vi "Teleop.vi"(10 "Match Info":T1={"Autonomous Elapsed Seconds"=0.0, "TeleOp Elapsed Seconds"=0.0, "Disabled Elapsed Seconds"=0.0, "Visited Autonomous"=FALSE, "Visited TeleOp"=FALSE, "Visited Disabled"=FALSE, "Autonomous Settings"={"Autonomous Style"=enum."Independent", "VI Refnum"=refnum}}, 11 "Call Context":T2) -> ()   [LabVIEW 2020]
doc: "This VI is called for each TeleOp packet received from the DS where the robot is not disabled. It is often used to read from the joysticks and update I/O or to update setpoints for timed control loops. It should complete and return within 20 milliseconds or it may miss DS packets."
uses:
  <vilib>/Rock Robotics/WPI/DriverStation/WPI_DriverStationDerivedRobotMode.ctl
  <vilib>/Rock Robotics/WPI/DriverStation/WPI_DriverStationMatch Info.ctl
  <vilib>/Rock Robotics/WPI/ThirdParty/Phoenix-LabVIEW/Motor Controller/Controls/CTRE_Phoenix_MotorControl_ControlMode.ctl
  <vilib>/Rock Robotics/WPI/ThirdParty/Phoenix-LabVIEW/Controls/CTRE_Phoenix_Params.ctl
  <vilib>/Rock Robotics/WPI/Utilities/WPI_GetSetVariantRefNum.vi
  <vilib>/Rock Robotics/Network Tables/NT Write Boolean Array.vi
  <vilib>/Rock Robotics/Network Tables/NT Write Numeric Array.vi
  <vilib>/Rock Robotics/Network Tables/NT Read Boolean.vi
  <vilib>/Rock Robotics/Network Tables/NT Read Number.vi
  <vilib>/Rock Robotics/WPI/Solenoid/Deprecated/WPI_SolenoidSetBool.vi
panel:
  out "encoder value":dbl
  out "Sample Slider 0":dbl(slide) scale=0.0..5.0
  out "Sample Boolean 1":bool
  out "Sample Boolean 0":bool
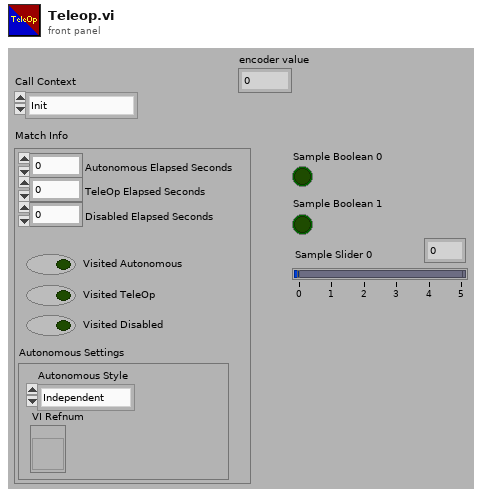
[diagram p1: front panel]
types:
  T1 = typedef "WPI_DriverStationMatch Info.ctl" = cluster{"Autonomous Elapsed Seconds":dbl, "TeleOp Elapsed Seconds":dbl, "Disabled Elapsed Seconds":dbl, "Visited Autonomous":bool, "Visited TeleOp":bool, "Visited Disabled":bool, "Autonomous Settings":cluster{"Autonomous Style":enum16{"Iterative", "Independent"}, "VI Refnum":refnum<vi>}}
  T2 = typedef "WPI_DriverStationDerivedRobotMode.ctl" = enum16{"Init", "Execute", "Stop"}
  T3 = typedef "CTRE_Phoenix_Params.ctl" = u16
  T4 = typedef "CTRE_Phoenix_MotorControl_ControlMode.ctl" = u16
  T5 = typedef "WPI_MotorControlDeviceRef.ctl" = cluster{"DeviceStatus":errorcluster, "Type":T6, "PWM":cluster{"PWM Channel":T7, "DeadBand":T8}, "CAN":cluster{"Device Number":u8, "SetOutput VI Ref":variant, "GetOutput VI Ref":variant, "Enable VI Ref":variant, "Disable VI Ref":variant, "Data":variant}, "Invert":bool, "DIO PWM":cluster{"PWM \"Enable\" Channel":T7, "DIOChannel":T9, "PWM Rate":dbl}}
  T6 = typedef "WPI_MotorControlType.ctl" = enum16{"PWM", "CAN", "DIO PWM"}
  T7 = typedef "FPGA_DIOPWMChannel.ctl" = enum8{"PWM 0", "PWM 1", "PWM 2", "PWM 3", "PWM 4", "PWM 5", "PWM 6", "PWM 7", "PWM 8", "PWM 9", "PWM MXP 0", "PWM MXP 1", "PWM MXP 2", "PWM MXP 3", "PWM MXP 4", "PWM MXP 5", "PWM MXP 6", "PWM MXP 7", "PWM MXP 8", "PWM MXP 9", "Invalid"}
  T8 = typedef "WPI_PWMDeadband.ctl" = cluster{"Name":string, "maxPositivePwm":i32, "minPositivePwm":i32, "centerPwm":i32, "maxNegativePwm":i32, "minNegativePwm":i32, "angularRange":u16}
  T9 = typedef "FPGA_DIOChannel.ctl" = enum8{"DIO 0", "DIO 1", "DIO 2", "DIO 3", "DIO 4", "DIO 5", "DIO 6", "DIO 7", "DIO 8", "DIO 9", "DIO MXP 0", "DIO MXP 1", "DIO MXP 2", "DIO MXP 3", "DIO MXP 4", "DIO MXP 5", "DIO MXP 6", "DIO MXP 7", "DIO MXP 8", "DIO MXP 9", "DIO MXP 10", "DIO MXP 11", "DIO MXP 12", "DIO MXP 13", "DIO MXP 14", "DIO MXP 15", "SPI Port CS1", "SPI Port CS2", "SPI Port CS3", "SPI Port MISO", "SPI Port MOSI", "Invalid"}
  T10 = typedef "WPI_JoystickDevRef.ctl" = cluster{"Device":T11}
  T11 = typedef "WPI_JoystickDeviceEnum.ctl" = enum16{"USB 0", "USB 1", "USB 2", "USB 3", "USB 4", "USB 5"}
  T12 = cluster{"Buttons[0]":bool, "Buttons[1]":bool, "Buttons[2]":bool, "Buttons[3]":bool, "Buttons[4]":bool, "Buttons[5]":bool, "Buttons[6]":bool, "Buttons[7]":bool, "Buttons[8]":bool}
  T13 = cluster{"Axes[0]":dbl, "Axes[1]":dbl, "Axes[2]":dbl, "Axes[3]":dbl, "Axes[4]":dbl, "Axes[5]":dbl, "Axes[6]":dbl, "Axes[7]":dbl, "Axes[8]":dbl}
  T14 = typedef "WPI_RobotDriveDevRef.ctl" = cluster{"DevStatus":errorcluster, "Motors[]":T5[], "Square Inputs":bool, "Max Output":dbl}
  T15 = typedef "WPI_SolenoidDevRef.ctl" = cluster{"DevStatus":errorcluster, "Pneumatics Control Module":u8, "Forward Solenoid Channel":T16, "Reverse Solenoid Channel":T16}
  T16 = typedef "WPI_SolenoidChannel.ctl" = enum8{"Solenoid 0", "Solenoid 1", "Solenoid 2", "Solenoid 3", "Solenoid 4", "Solenoid 5", "Solenoid 6", "Solenoid 7", "Solenoid 8", "Solenoid 9", "Solenoid 10", "Solenoid 11", "Solenoid 12", "Solenoid 13", "Solenoid 14", "Solenoid 15", "Invalid"}
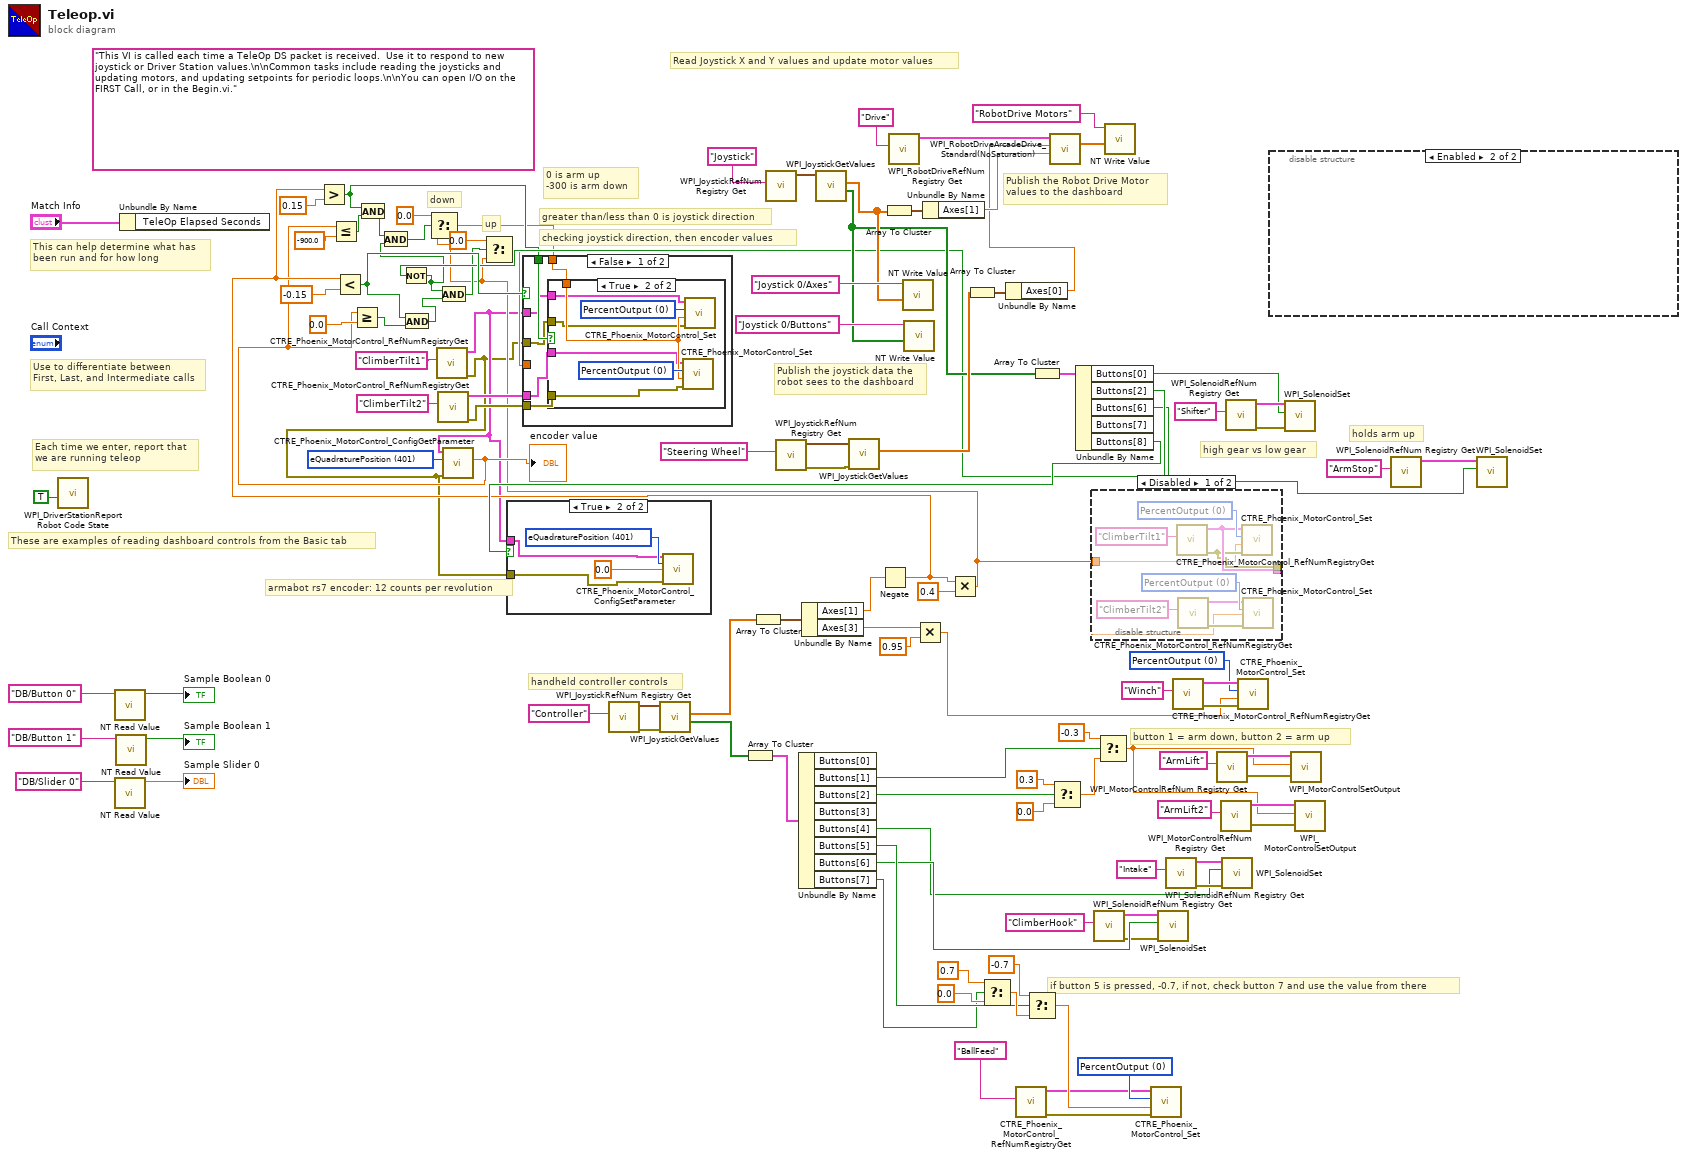
[diagram p0: block diagram]
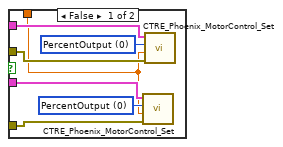
[diagram p3: hidden frame]
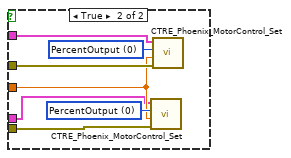
[diagram p4: hidden frame]
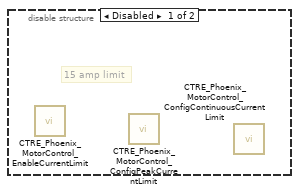
[diagram p6: hidden frame]
diagram:
  w22 = T3 401 items=["eOnBoot_BrakeMode"=31, "eQuadFilterEn"=91, "eClearPositionOnIdx"=100, "eQuadIdxPolarity"=108, "eMotionProfileHasUnderrunErr"=119, "eMotionProfileTrajectoryPointDurationMs"=120, "eMotionProfileTrajectoryInterpolDis"=121, "eClearPosOnLimitF"=144, "eClearPosOnLimitR"=145, "eYawOffset"=160, "eCompassOffset"=161, "eBetaGain"=162, "eEnableCompassFustion"=163, "eGyroNoMotionCal"=164, "eEnterCalibration"=165, "eFusedHeadingOffset"=166, "eStatusFrameRate"=169, "eAccumZ"=170, "eTempCompDisable"=171, "eMotionMeas_tap_threshX"=172, "eMotionMeas_tap_threshY"=173, "eMotionMeas_tap_threshZ"=174, "eMotionMeas_tap_count"=175, "eMotionMeas_tap_time"=176, "eMotionMeas_tap_time_multi"=177, "eMotionMeas_shake_reject_thresh"=178, "eMotionMeas_shake_reject_time"=179, "eMotionMeas_shake_reject_timeout"=180, "eStatusFramePeriod"=300, "eOpenLoopRamp"=301, "eClosedLoopRamp"=302, "eNeutralDeadband"=303, "ePeakPosOutput"=305, "eNominalPosOutput"=306, "ePeakNegOutput"=307, "eNominalNegOutput"=308, "eProfileParamSlot_P"=310, "eProfileParamSlot_I"=311, "eProfileParamSlot_D"=312, "eProfileParamSlot_F"=313, "eProfileParamSlot_IZone"=314, "eProfileParamSlot_AllowableErr"=315, "eProfileParamSlot_MaxIAccum"=316, "eProfileParamSlot_PeakOutput"=317, "eClearPositionOnLimitF"=320, "eClearPositionOnLimitR"=321, "eClearPositionOnQuadIdx"=322, "eSampleVelocityPeriod"=325, "eSampleVelocityWindow"=326, "eFeedbackSensorType"=330, "eSelectedSensorPosition"=331, "eFeedbackNotContinuous"=332, "eRemoteSensorSource"=333, "eRemoteSensorDeviceID"=334, "eSensorTerm"=335, "eRemoteSensorClosedLoopDisableNeutralOnLOS"=336, "ePIDLoopPolarity"=337, "ePIDLoopPeriod"=338, "eSelectedSensorCoefficient"=339, "eForwardSoftLimitThreshold"=340, "eReverseSoftLimitThreshold"=341, "eForwardSoftLimitEnable"=342, "eReverseSoftLimitEnable"=343, "eNominalBatteryVoltage"=350, "eBatterVoltageFilterSize"=351, "eContinuousCurrentLimitAmps"=360, "eContinuousCurrentLimitMs"=361, "ePeakCurrentLimitAmps"=362, "eCurrEnable"=363, "eCurrThres_Ms"=364, "eClosedLoopIAccum"=370, "eCustomParam"=380, "eStickyFaults"=390, "eAnalogPosition"=400, "eQuadraturePosition"=401, "ePulseWidthPosition"=402, "eIntegratedSensor"=403, "eMotMag_Accel"=410, "eMotMag_VelCruise"=411, "eMotMag_SCurveLevel"=412, "eLimitSwitchSource"=421, "eLimitSwitchNormClosedAndDis"=422, "eLimitSwitchDisabledNeutralOnLOS"=423, "eLimitSwitchRemoteDevID"=424, "eSoftLimitDisabledNeutralOnLOS"=425, "ePulseWidthPeriod_EdgesPerRot"=430, "ePulseWidthPeriod_FilterWindowSz"=431, "eUnitString"=442, "eFeedbackTimeBase"=443, "eDefaultConfig"=500, "eFastWriteCount"=501, "eWriteCount"=502, "eReserved1"=555, "eMotorCommutation"=650, "eSensorInitStrategy"=700, "eSensorDirection"=701, "eMagnetOffset"=702, "eSensorSync"=703, "eAbsSensorRange"=704, "eChangeCompassUse"=800, "eRestartKalman"=801, "eAccNoiseAmplificationGain"=802, "eMagNoiseAmplificationGain"=803, "eGyrNoiseAmplificationGain"=804, "eMaxAccKg"=805, "eMaxMagKg"=806, "eGyroBias"=807, "eAccelOffsets"=808, "eMagCal"=809, "eMagCalSlot"=810, "eMagCalRunning"=811, "eGyrResolution"=812, "eAccelKalmanBiasGain"=813, "eMagKalmanBiasGain"=814, "eTempCalRunning"=815, "eApplyTempCal"=816, "eClearTempCal"=817, "eDontRunThermComp"=818, "eChangeHeatOutput"=819, "eSetNoMotionCalDisable"=820, "eClearMagCal"=821, "eSetGyrSensitivity"=822, "eSetVsenseScalar"=823, "eConfigMountPoseYaw"=824, "eConfigMountPosePitch"=825, "eConfigMountPoseRoll"=826, "eConfigAccelScalar"=827, "eLEDStripType"=900, "eLossOfSignalBehavior"=901, "eBrightnessCoefficient"=902, "eStatusLedState"=903, "eVBatOutput"=904] ("Parameter")
  w48 = T4 0 items=["PercentOutput"=0, "Position"=1, "Velocity"=2, "Current"=3, "Follower"=5, "MotionProfile"=6, "MotionMagic"=7, "MotionProfileArc"=10, "Disabled"=15] ("Control Mode")
  w79 = T4 0 items=["PercentOutput"=0, "Position"=1, "Velocity"=2, "Current"=3, "Follower"=5, "MotionProfile"=6, "MotionMagic"=7, "MotionProfileArc"=10, "Disabled"=15] ("Control Mode")
  (unwired) "This VI is called each time a TeleOp DS packet is received.  Use it to respond to new joystick or Driver Station values.\n\nCommon tasks include reading the joysticks and updating motors, and updating setpoints for periodic loops.\n\nYou can open I/O on the FIRST Call, or in the Begin.vi."
  # "down"
  # "up"
  # "checking joystick direction, then encoder values"
  # "greater than/less than 0 is joystick direction"
  # "0 is arm up\n-300 is arm down"
  # "armabot rs7 encoder: 12 counts per revolution"
  # "holds arm up"
  # "button 1 = arm down, button 2 = arm up"
  # "if button 5 is pressed, -0.7, if not, check button 7 and use the value from there"
  # "high gear vs low gear"
  # "handheld controller controls"
  # "These are examples of reading dashboard controls from the Basic tab"
  # "Publish the Robot Drive Motor\nvalues to the dashboard"
  # "Publish the joystick data the\nrobot sees to the dashboard"
  # "Each time we enter, report that\nwe are running teleop"
  # "Use to differentiate between\nFirst, Last, and Intermediate calls"
  # "This can help determine what has\nbeen run and for how long"
  # "Read Joystick X and Y values and update motor values"
  n1 = call <vilib>:"WPI_DriverStationReport Robot Code State.vi"("TeleOp"=TRUE ("Autonomous")) -> ()  [unwired: 10 in, 1 out]
  n2 = call-poly <vilib>:"NT Read Value.vi"("Name"="DB/Button 0" ("refnum name")) -> ("Boolean"=→"Sample Boolean 0":bool)  [unwired: 9 in, 1 out]
  n3 = call-poly <vilib>:"NT Read Value.vi"("Name"="DB/Slider 0" ("refnum name")) -> ("Numeric"=→"Sample Slider 0":dbl)  [unwired: 9 in, 1 out]
  n4 = call-poly <vilib>:"NT Read Value.vi"("Name"="DB/Button 1" ("refnum name")) -> ("Boolean"=→"Sample Boolean 1":bool)  [unwired: 9 in, 1 out]
  n5 = Unbundle By Name("Match Info") -> ()  [unwired: 1 out]
  n6 = call <vilib>:"CTRE_Phoenix_MotorControl_RefNumRegistryGet.vi"("refnum name"="ClimberTilt1") -> ("error out"=w1:errorcluster, "PhoenixMotorControlDevRef"=w2:T5)  [unwired: 9 in]
  n7 = call <vilib>:"CTRE_Phoenix_MotorControl_RefNumRegistryGet.vi"("refnum name"="ClimberTilt2") -> ("error out"=w20:errorcluster, "PhoenixMotorControlDevRef"=w21:T5)  [unwired: 9 in]
  n8 = call <vilib>:"CTRE_Phoenix_MotorControl_ConfigGetParameter.vi"("error in (no error)"=w1, "Parameter"=w22, "PhoenixMotorControlDevRef"=w2) -> ("value"=w15:dbl)  [unwired: 6 in, 2 out]
  "encoder value" <- w15
  n9 = Less Or Equal?(x=w15, y=-900.0) -> (x <= y?=w12:bool)
  n10 = Greater Or Equal?(x=w15, y=0.0) -> (x >= y?=w26:bool)
  n11 = call <vilib>:"WPI_JoystickRefNum Registry Get.vi"("refnum name"="Controller") -> ("error out"=w86:errorcluster, "JoystickDevRef"=w85:T10)  [unwired: 9 in]
  n12 = call <vilib>:"WPI_JoystickGetValues.vi"("error in (no error)"=w86, "JoystickDevRef"=w85) -> ("Buttons"=w83:bool[], "Axes"=w70:dbl[])  [unwired: 5 in, 3 out]
  n13 = Array To Cluster(array=w83) -> (cluster=w82:T12)
  n14 = Array To Cluster(array=w70) -> (cluster=w69:T13)
  n15 = call <vilib>:"WPI_JoystickRefNum Registry Get.vi"("refnum name"="Joystick") -> ("JoystickDevRef"=w107:T10)  [unwired: 1 in, 9 out]
  n16 = call <vilib>:"WPI_JoystickRefNum Registry Get.vi"("refnum name"="Steering Wheel") -> ("error out"=w94:errorcluster, "JoystickDevRef"=w95:T10)  [unwired: 9 in]
  n17 = Unbundle By Name(w82) -> ("Buttons[1]"=w68:bool, "Buttons[2]"=w66:bool, "Buttons[4]"=w39:bool, "Buttons[5]"=w59:bool, "Buttons[6]"=w43:bool, "Buttons[7]"=w58:bool)  [unwired: 2 out]
  n18 = Unbundle By Name(w69) -> ("Axes[1]"=w33:dbl, "Axes[3]"=w46:dbl)
  n19 = call <vilib>:"WPI_JoystickGetValues.vi"("JoystickDevRef"=w107) -> ("Buttons"=w57:bool[], "Axes"=w92:dbl[])  [unwired: 6 in, 3 out]
  n20 = call <vilib>:"WPI_JoystickGetValues.vi"("error in (no error)"=w94, "JoystickDevRef"=w95) -> ("Axes"=w90:dbl[])  [unwired: 5 in, 4 out]
  n21 = Negate(x=w33) -> (-x=w17:dbl)
  n22 = Greater?(x=w17, y=0.15) -> (0:w13:bool)
  n23 = Less?(x=w17, y=-0.15) -> (x < y?=w19:bool)
  n24 = And(x=w13, y=w12) -> (x .and. y?=w11:bool)
  n25 = And(x=w19, y=w26) -> (x .and. y?=w25:bool)
  n26 = Array To Cluster(array=w92) -> (cluster=w91:T13)
  n27 = call <vilib>:"WPI_RobotDriveRefNum Registry Get.vi"("refnum name"="Drive") -> ("RobotDriveDevRef"=w109:T14)  [unwired: 1 in, 9 out]
  n28 = call-poly <vilib>:"NT Write Value.vi"("Numeric Array"=w92, "Name"="Joystick 0/Axes") -> ()  [unwired: 9 in, 1 out]
  n29 = call-poly <vilib>:"NT Write Value.vi"("Boolean Array"=w57, "Name"="Joystick 0/Buttons") -> ()  [unwired: 9 in, 1 out]
  n30 = Multiply(x=w46, y=0.95) -> (x*y=w44:dbl)
  n31 = Unbundle By Name(w91) -> ("Axes[1]"=w88:dbl)
  n32 = Multiply(x=w17, y=0.4) -> (x*y=w4:dbl)
  n33 = Array To Cluster(array=w90) -> (cluster=w89:T13)
  n34 = Select(t=0.7, s=w58, f=0.0) -> (s? t:f=w77:dbl)
  n35 = Unbundle By Name(w89) -> ("Axes[0]"=w87:dbl)
  n36 = call <vilib>:"CTRE_Phoenix_MotorControl_RefNumRegistryGet.vi"("refnum name"="BallFeed") -> ("error out"=w74:errorcluster, "PhoenixMotorControlDevRef"=w75:T5)  [unwired: 9 in]
  n37 = Select(t=-0.7, s=w59, f=w77) -> (s? t:f=w76:dbl)
  n38 = Array To Cluster(array=w57) -> (cluster=w56:T12)
  n39 = call <vilib>:"WPI_RobotDriveArcadeDrive_Standard(NoSaturation).vi"("Y axis value"=w88, "X axis value"=w87, "RobotDriveDevRef"=w109) -> ("Motor Values"=w97:dbl[])  [unwired: 1 in, 7 out]
  n40 = Select(t=0.3, s=w66, f=0.0) -> (s? t:f=w65:dbl)
  n41 = Unbundle By Name(w56) -> ("Buttons[0]"=w53:bool, "Buttons[2]"=w30:bool, "Buttons[6]"=w18:bool, "Buttons[8]"=w29:bool)  [unwired: 1 out]
  n42 = Not(x=w18) -> (.not. x?=w10:bool)
  n43 = And(x=w11, y=w10) -> (x .and. y?=w6:bool)
  n44 = Select(t=0.0, s=w6, f=w4) -> (s? t:f=w3:dbl)
  n45 = And(x=w10, y=w25) -> (x .and. y?=w9:bool)
  n46 = Select(t=0.0, s=w9, f=w4) -> (s? t:f=w7:dbl)
  n47 = case shown="True" w29 {
    tunnel: w2 -> [_ w113]
    tunnel: w1 -> [_ w112]
    frame False {
    }
    frame True {
      w115 = T3 401 items=["eOnBoot_BrakeMode"=31, "eQuadFilterEn"=91, "eClearPositionOnIdx"=100, "eQuadIdxPolarity"=108, "eMotionProfileHasUnderrunErr"=119, "eMotionProfileTrajectoryPointDurationMs"=120, "eMotionProfileTrajectoryInterpolDis"=121, "eClearPosOnLimitF"=144, "eClearPosOnLimitR"=145, "eYawOffset"=160, "eCompassOffset"=161, "eBetaGain"=162, "eEnableCompassFustion"=163, "eGyroNoMotionCal"=164, "eEnterCalibration"=165, "eFusedHeadingOffset"=166, "eStatusFrameRate"=169, "eAccumZ"=170, "eTempCompDisable"=171, "eMotionMeas_tap_threshX"=172, "eMotionMeas_tap_threshY"=173, "eMotionMeas_tap_threshZ"=174, "eMotionMeas_tap_count"=175, "eMotionMeas_tap_time"=176, "eMotionMeas_tap_time_multi"=177, "eMotionMeas_shake_reject_thresh"=178, "eMotionMeas_shake_reject_time"=179, "eMotionMeas_shake_reject_timeout"=180, "eStatusFramePeriod"=300, "eOpenLoopRamp"=301, "eClosedLoopRamp"=302, "eNeutralDeadband"=303, "ePeakPosOutput"=305, "eNominalPosOutput"=306, "ePeakNegOutput"=307, "eNominalNegOutput"=308, "eProfileParamSlot_P"=310, "eProfileParamSlot_I"=311, "eProfileParamSlot_D"=312, "eProfileParamSlot_F"=313, "eProfileParamSlot_IZone"=314, "eProfileParamSlot_AllowableErr"=315, "eProfileParamSlot_MaxIAccum"=316, "eProfileParamSlot_PeakOutput"=317, "eClearPositionOnLimitF"=320, "eClearPositionOnLimitR"=321, "eClearPositionOnQuadIdx"=322, "eSampleVelocityPeriod"=325, "eSampleVelocityWindow"=326, "eFeedbackSensorType"=330, "eSelectedSensorPosition"=331, "eFeedbackNotContinuous"=332, "eRemoteSensorSource"=333, "eRemoteSensorDeviceID"=334, "eSensorTerm"=335, "eRemoteSensorClosedLoopDisableNeutralOnLOS"=336, "ePIDLoopPolarity"=337, "ePIDLoopPeriod"=338, "eSelectedSensorCoefficient"=339, "eForwardSoftLimitThreshold"=340, "eReverseSoftLimitThreshold"=341, "eForwardSoftLimitEnable"=342, "eReverseSoftLimitEnable"=343, "eNominalBatteryVoltage"=350, "eBatterVoltageFilterSize"=351, "eContinuousCurrentLimitAmps"=360, "eContinuousCurrentLimitMs"=361, "ePeakCurrentLimitAmps"=362, "eCurrEnable"=363, "eCurrThres_Ms"=364, "eClosedLoopIAccum"=370, "eCustomParam"=380, "eStickyFaults"=390, "eAnalogPosition"=400, "eQuadraturePosition"=401, "ePulseWidthPosition"=402, "eIntegratedSensor"=403, "eMotMag_Accel"=410, "eMotMag_VelCruise"=411, "eMotMag_SCurveLevel"=412, "eLimitSwitchSource"=421, "eLimitSwitchNormClosedAndDis"=422, "eLimitSwitchDisabledNeutralOnLOS"=423, "eLimitSwitchRemoteDevID"=424, "eSoftLimitDisabledNeutralOnLOS"=425, "ePulseWidthPeriod_EdgesPerRot"=430, "ePulseWidthPeriod_FilterWindowSz"=431, "eUnitString"=442, "eFeedbackTimeBase"=443, "eDefaultConfig"=500, "eFastWriteCount"=501, "eWriteCount"=502, "eReserved1"=555, "eMotorCommutation"=650, "eSensorInitStrategy"=700, "eSensorDirection"=701, "eMagnetOffset"=702, "eSensorSync"=703, "eAbsSensorRange"=704, "eChangeCompassUse"=800, "eRestartKalman"=801, "eAccNoiseAmplificationGain"=802, "eMagNoiseAmplificationGain"=803, "eGyrNoiseAmplificationGain"=804, "eMaxAccKg"=805, "eMaxMagKg"=806, "eGyroBias"=807, "eAccelOffsets"=808, "eMagCal"=809, "eMagCalSlot"=810, "eMagCalRunning"=811, "eGyrResolution"=812, "eAccelKalmanBiasGain"=813, "eMagKalmanBiasGain"=814, "eTempCalRunning"=815, "eApplyTempCal"=816, "eClearTempCal"=817, "eDontRunThermComp"=818, "eChangeHeatOutput"=819, "eSetNoMotionCalDisable"=820, "eClearMagCal"=821, "eSetGyrSensitivity"=822, "eSetVsenseScalar"=823, "eConfigMountPoseYaw"=824, "eConfigMountPosePitch"=825, "eConfigMountPoseRoll"=826, "eConfigAccelScalar"=827, "eLEDStripType"=900, "eLossOfSignalBehavior"=901, "eBrightnessCoefficient"=902, "eStatusLedState"=903, "eVBatOutput"=904] ("Parameter")
      n48 = call <vilib>:"CTRE_Phoenix_MotorControl_ConfigSetParameter.vi"("PhoenixMotorControlDevRef"=w113, "Parameter"=w115, "value"=0.0, "error in (no error)"=w112) -> ()  [unwired: 10 in, 2 out]
    }
  }
  n49 = case shown="False" w19 {
    tunnel: w7 -> [_ w138]
    tunnel: w2 -> [w119 w141]
    tunnel: w1 -> [w118 w140]
    tunnel: w21 -> [w117 w137]
    tunnel: w20 -> [w116 w136]
    tunnel: w13 -> [w121 _]
    tunnel: w3 -> [w120 _]
    frame False {
      n50 = case shown="True" w121 {
        tunnel: w120 -> [w122 w133]
        tunnel: w119 -> [w126 w132]
        tunnel: w118 -> [w125 w131]
        tunnel: w117 -> [w124 w130]
        tunnel: w116 -> [w123 w129]
        frame False {
          w127 = T4 0 items=["PercentOutput"=0, "Position"=1, "Velocity"=2, "Current"=3, "Follower"=5, "MotionProfile"=6, "MotionMagic"=7, "MotionProfileArc"=10, "Disabled"=15] ("Control Mode")
          w128 = T4 0 items=["PercentOutput"=0, "Position"=1, "Velocity"=2, "Current"=3, "Follower"=5, "MotionProfile"=6, "MotionMagic"=7, "MotionProfileArc"=10, "Disabled"=15] ("Control Mode")
          n51 = call <vilib>:"CTRE_Phoenix_MotorControl_Set.vi"("error in (no error)"=w123, "Output"=w122, "Control Mode"=w127, "PhoenixMotorControlDevRef"=w124) -> ()  [unwired: 6 in, 2 out]
          n52 = call <vilib>:"CTRE_Phoenix_MotorControl_Set.vi"("error in (no error)"=w125, "Output"=w122, "Control Mode"=w128, "PhoenixMotorControlDevRef"=w126) -> ()  [unwired: 6 in, 2 out]
        }
        frame True {
          w134 = T4 0 items=["PercentOutput"=0, "Position"=1, "Velocity"=2, "Current"=3, "Follower"=5, "MotionProfile"=6, "MotionMagic"=7, "MotionProfileArc"=10, "Disabled"=15] ("Control Mode")
          w135 = T4 0 items=["PercentOutput"=0, "Position"=1, "Velocity"=2, "Current"=3, "Follower"=5, "MotionProfile"=6, "MotionMagic"=7, "MotionProfileArc"=10, "Disabled"=15] ("Control Mode")
          n53 = call <vilib>:"CTRE_Phoenix_MotorControl_Set.vi"("error in (no error)"=w129, "Output"=w133, "Control Mode"=w134, "PhoenixMotorControlDevRef"=w130) -> ()  [unwired: 6 in, 2 out]
          n54 = call <vilib>:"CTRE_Phoenix_MotorControl_Set.vi"("error in (no error)"=w131, "Output"=w133, "Control Mode"=w135, "PhoenixMotorControlDevRef"=w132) -> ()  [unwired: 6 in, 2 out]
        }
      }
    }
    frame True {
      w139 = T4 0 items=["PercentOutput"=0, "Position"=1, "Velocity"=2, "Current"=3, "Follower"=5, "MotionProfile"=6, "MotionMagic"=7, "MotionProfileArc"=10, "Disabled"=15] ("Control Mode")
      w142 = T4 0 items=["PercentOutput"=0, "Position"=1, "Velocity"=2, "Current"=3, "Follower"=5, "MotionProfile"=6, "MotionMagic"=7, "MotionProfileArc"=10, "Disabled"=15] ("Control Mode")
      n55 = call <vilib>:"CTRE_Phoenix_MotorControl_Set.vi"("error in (no error)"=w136, "Output"=w138, "Control Mode"=w139, "PhoenixMotorControlDevRef"=w137) -> ()  [unwired: 6 in, 2 out]
      n56 = call <vilib>:"CTRE_Phoenix_MotorControl_Set.vi"("error in (no error)"=w140, "Output"=w138, "Control Mode"=w142, "PhoenixMotorControlDevRef"=w141) -> ()  [unwired: 6 in, 2 out]
    }
  }
  n57 = disable-structure shown="Disabled" {
    disable-tunnel: [w145 _] -> _
    disable-tunnel: [w144 _] -> _
    disable-tunnel: w4 -> [w143 _]
    frame Disabled {
      w148 = T4 0 items=["PercentOutput"=0, "Position"=1, "Velocity"=2, "Current"=3, "Follower"=5, "MotionProfile"=6, "MotionMagic"=7, "MotionProfileArc"=10, "Disabled"=15] ("Control Mode")
      w149 = T4 0 items=["PercentOutput"=0, "Position"=1, "Velocity"=2, "Current"=3, "Follower"=5, "MotionProfile"=6, "MotionMagic"=7, "MotionProfileArc"=10, "Disabled"=15] ("Control Mode")
      n58 = call <vilib>:"CTRE_Phoenix_MotorControl_RefNumRegistryGet.vi"("refnum name"="ClimberTilt1") -> ("error out"=w144:errorcluster, "PhoenixMotorControlDevRef"=w145:T5)  [unwired: 9 in]
      n59 = call <vilib>:"CTRE_Phoenix_MotorControl_RefNumRegistryGet.vi"("refnum name"="ClimberTilt2") -> ("error out"=w146:errorcluster, "PhoenixMotorControlDevRef"=w147:T5)  [unwired: 9 in]
      n60 = call <vilib>:"CTRE_Phoenix_MotorControl_Set.vi"("error in (no error)"=w144, "Output"=w143, "Control Mode"=w149, "PhoenixMotorControlDevRef"=w145) -> ()  [unwired: 6 in, 2 out]
      n61 = call <vilib>:"CTRE_Phoenix_MotorControl_Set.vi"("error in (no error)"=w146, "Output"=w143, "Control Mode"=w148, "PhoenixMotorControlDevRef"=w147) -> ()  [unwired: 6 in, 2 out]
    }
    frame Enabled {
    }
  }
  n62 = call <vilib>:"WPI_SolenoidRefNum Registry Get.vi"("refnum name"="ClimberHook") -> ("error out"=w41:errorcluster, "SolenoidDevRef"=w42:T15)  [unwired: 9 in]
  n63 = Select(t=-0.3, s=w68, f=w65) -> (s? t:f=w34:dbl)
  n64 = call-poly <vilib>:"NT Write Value.vi"("Numeric Array"=w97, "Name"="RobotDrive Motors") -> ()  [unwired: 9 in, 1 out]
  n65 = call <vilib>:"CTRE_Phoenix_MotorControl_Set.vi"("error in (no error)"=w74, "Output"=w76, "Control Mode"=w79, "PhoenixMotorControlDevRef"=w75) -> ()  [unwired: 6 in, 2 out]
  n66 = call-poly <vilib>:"WPI_SolenoidSet.vi"("error in (no error)"=w41, "Value"=w43, "SolenoidDevRef"=w42) -> ()  [unwired: 7 in, 2 out]
  n67 = call <vilib>:"WPI_SolenoidRefNum Registry Get.vi"("refnum name"="Intake") -> ("error out"=w62:errorcluster, "SolenoidDevRef"=w61:T15)  [unwired: 9 in]
  n68 = call <vilib>:"CTRE_Phoenix_MotorControl_RefNumRegistryGet.vi"("refnum name"="Winch") -> ("error out"=w50:errorcluster, "PhoenixMotorControlDevRef"=w51:T5)  [unwired: 9 in]
  n69 = call <vilib>:"WPI_MotorControlRefNum Registry Get.vi"("refnum name"="ArmLift") -> ("error out"=w71:errorcluster, "MotorControlDevRef"=w72:T5)  [unwired: 9 in]
  n70 = call <vilib>:"WPI_MotorControlRefNum Registry Get.vi"("refnum name"="ArmLift2") -> ("error out"=w38:errorcluster, "MotorControlDevRef"=w37:T5)  [unwired: 9 in]
  n71 = call-poly <vilib>:"WPI_SolenoidSet.vi"("error in (no error)"=w62, "Value"=w39, "SolenoidDevRef"=w61) -> ()  [unwired: 7 in, 2 out]
  n72 = call <vilib>:"WPI_SolenoidRefNum Registry Get.vi"("refnum name"="Shifter") -> ("error out"=w54:errorcluster, "SolenoidDevRef"=w55:T15)  [unwired: 9 in]
  n73 = call <vilib>:"CTRE_Phoenix_MotorControl_Set.vi"("error in (no error)"=w50, "Output"=w44, "Control Mode"=w48, "PhoenixMotorControlDevRef"=w51) -> ()  [unwired: 6 in, 2 out]
  n74 = disable-structure shown="Enabled" {
    frame Disabled {
      # "15 amp limit"
      n75 = call <vilib>:"CTRE_Phoenix_MotorControl_EnableCurrentLimit.vi"() -> ()  [unwired: 10 in, 2 out]
      n76 = call <vilib>:"CTRE_Phoenix_MotorControl_ConfigPeakCurrentLimit.vi"() -> ()  [unwired: 10 in, 2 out]
      n77 = call <vilib>:"CTRE_Phoenix_MotorControl_ConfigContinuousCurrentLimit.vi"() -> ()  [unwired: 10 in, 2 out]
    }
    frame Enabled {
    }
  }
  n78 = call-poly <vilib>:"WPI_SolenoidSet.vi"("error in (no error)"=w54, "Value"=w53, "SolenoidDevRef"=w55) -> ()  [unwired: 7 in, 2 out]
  n79 = call <vilib>:"WPI_MotorControlSetOutput.vi"("error in (no error)"=w71, "Output"=w34, "MotorControlDevRef"=w72) -> ()  [unwired: 6 in, 3 out]
  n80 = call <vilib>:"WPI_MotorControlSetOutput.vi"("error in (no error)"=w38, "Output"=w34, "MotorControlDevRef"=w37) -> ()  [unwired: 6 in, 3 out]
  n81 = call <vilib>:"WPI_SolenoidRefNum Registry Get.vi"("refnum name"="ArmStop") -> ("SolenoidDevRef"=w31:T15)  [unwired: 9 in, 1 out]
  n82 = call-poly <vilib>:"WPI_SolenoidSet.vi"("Value"=w30, "SolenoidDevRef"=w31) -> ()  [unwired: 8 in, 2 out]
